vi "Create AnntList for Graph.vi"(8 "Internal Channel Toggle List":string[](array[string]), 9 "Internal Channel Name List":string[](array[string]), 10 "Label Precision":i32, 11 "Graph Input":cluster{timestamp[], dbl[]}[](array[cluster])) -> (0 "Last Measurements":string[][](array[string]), 3 "AnntList Input":T1(array[cluster]))   [LabVIEW 2023]
uses:
  8632bbc3-2c05-c44b-aaba-464b769b071b.vi
  <vilib>/Array/Sort 2D Array - Pop Stack.vi
  <vilib>/Array/Sort 2D Array - Push Stack.vi
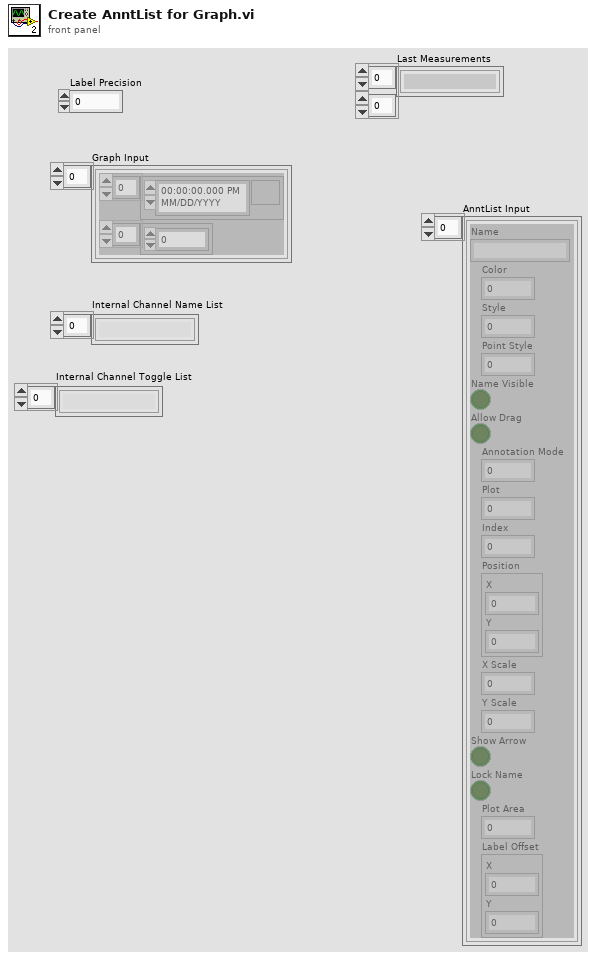
[diagram p1: front panel]
types:
  T1 = cluster{"Name":string, "Color":u32, "Style":u8, "Point Style":u8, "Name Visible":bool, "Allow Drag":bool, "Annotation Mode":u32, "Plot":i32, "Index":i32, "Position":cluster{"X":dbl, "Y":dbl}, "X Scale":u32, "Y Scale":u32, "Show Arrow":bool, "Lock Name":bool, "Plot Area":i32, "Label Offset":cluster{"X":dbl, "Y":dbl}}[]
  T2 = cluster{"Name":string, "Color":i32, "Style":u8, "Point Style":u8, "Name Visible":bool, "Allow Drag":bool, "Annotation Mode":u32, "Plot":i32, "Index":i32, "Position":cluster{"X":dbl, "Y":dbl}, "X Scale":u32, "Y Scale":u32, "Show Arrow":bool, "Lock Name":bool, "Plot Area":i32, "Label Offset":cluster{"X":i32, "Y":i32}}
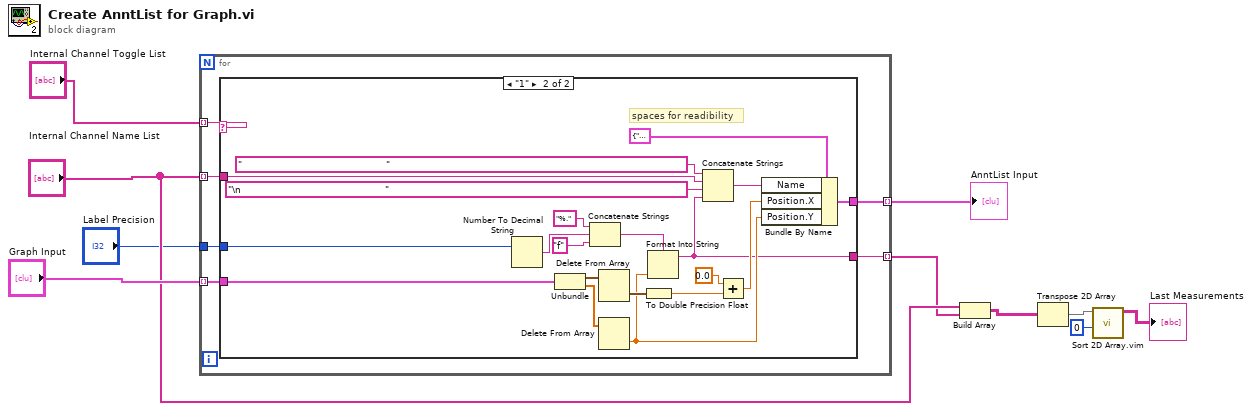
[diagram p0: block diagram]
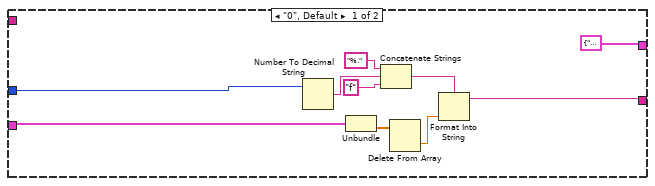
[diagram p2: hidden frame]
diagram:
  n1 = for {
    tunnel: "Graph Input" -> [w16] mode=indexing
    tunnel: [w15] -> w9 mode=indexing
    tunnel: "Internal Channel Name List" -> [w14] mode=indexing
    tunnel: [w13] -> w7 mode=indexing
    tunnel: "Internal Channel Toggle List" -> [w12] mode=indexing
    tunnel: "Label Precision" -> [w11]
    n2 = case shown="\"1\"" w12 {
      tunnel: w16 -> [w19 w45]
      tunnel: [T2 {"Name"="", "Color"=16777215, "Style"=0, "Point Style"=0, "Name Visible"=TRUE, "Allow Drag"=TRUE, "Annotation Mode"=0, "Plot"=0, "Index"=0, "Position"={"X"=0.0, "Y"=0.0}, "X Scale"=0, "Y Scale"=0, "Show Arrow"=FALSE, "Lock Name"=FALSE, "Plot Area"=0, "Label Offset"={"X"=0, "Y"=0}} w41] -> w15
      tunnel: w14 -> [_ w31]
      tunnel: [w20 w28] -> w13
      tunnel: w11 -> [w18 w27]
      frame "0", Default {
        n3 = Number To Decimal String(number=w18) -> (decimal integer string=w22:string)  [unwired: 1 in]
        n4 = Unbundle(w19) -> (w26:dbl[])  [unwired: 1 out]
        n5 = Concatenate Strings("%." ("string"), w22, "f" ("string")) -> (w21:string)
        n6 = Delete From Array(array=w26) -> (deleted portion=w25:dbl)  [unwired: 2 in, 1 out]
        n7 = Format Into String(format string=w21, w25) -> (resulting string=w20:string)  [unwired: 2 in, 1 out]
      }
      frame "1" {
        # "spaces for readibility"
        n8 = Number To Decimal String(number=w27) -> (decimal integer string=w37:string)  [unwired: 1 in]
        n9 = Unbundle(w45) -> (w44:timestamp[], w43:dbl[])
        n10 = Concatenate Strings("%." ("string"), w37, "f" ("string")) -> (w36:string)
        n11 = Delete From Array(array=w44) -> (deleted portion=w42:timestamp)  [unwired: 2 in, 1 out]
        n12 = Delete From Array(array=w43) -> (deleted portion=w40:dbl)  [unwired: 2 in, 1 out]
        n13 = To Double Precision Float(number=w42) -> (double precision float=w34:dbl)
        n14 = Format Into String(format string=w36, w40) -> (resulting string=w28:string)  [unwired: 2 in, 1 out]
        n15 = Concatenate Strings("                                                " ("string"), w31, "\n                                                " ("string"), w28) -> (w30:string)
        n16 = Add(x=0.0, y=w34) -> (x+y=w35:dbl)
        n17 = Bundle By Name(cluster=T2 {"Name"="", "Color"=16777215, "Style"=0, "Point Style"=0, "Name Visible"=TRUE, "Allow Drag"=TRUE, "Annotation Mode"=0, "Plot"=0, "Index"=0, "Position"={"X"=0.0, "Y"=0.0}, "X Scale"=0, "Y Scale"=0, "Show Arrow"=FALSE, "Lock Name"=FALSE, "Plot Area"=0, "Label Offset"={"X"=0, "Y"=0}}, "Name"=w30, "Position.X"=w35, "Position.Y"=w40) -> (w41:T2)
      }
    }
  }
  "AnntList Input" <- w9
  n18 = Build Array("Internal Channel Name List", w7) -> (w6:string[][])
  n19 = Transpose 2D Array(2D array=w6) -> (transposed array=w5:string[][])
  n20 = call "Sort 2D Array.vim"("index"=0, "2D array"=w5) -> ("sorted 2D array"=→"Last Measurements":string[][])  [unwired: 8 in, 1 out]
